vi "CreateSelfReference.vi"(8 "error in (no error)":errorcluster, 11 "XYStage":refnum<class "XYStage.lvclass">) -> (0 "error out":errorcluster, 3 "XYStage out":refnum<class "XYStage.lvclass">)   [LabVIEW 2013, in "XYStage.lvclass"]
doc: "JKI State Machine Objects (SMO) 1.0.0.5\nJKI - JKI\nCopyright (c) 2016, JKI"
uses:
  XYStage.lvclass
  <vilib>/JKI/JKI SMO/SMO/SMO.lvclass
panel:
  # "For instructions on how to use the JKI State Machine Objects, examples and video tutorials, visit:\nhttp://jki.net/state-machine-objects/\n\nJKI State Machine Objects™\nhttp://jki.net/state-machine-objects/\nCopyright (C) 2005-2015, JKI <info@jki.net>\nALL RIGHTS RESERVED"
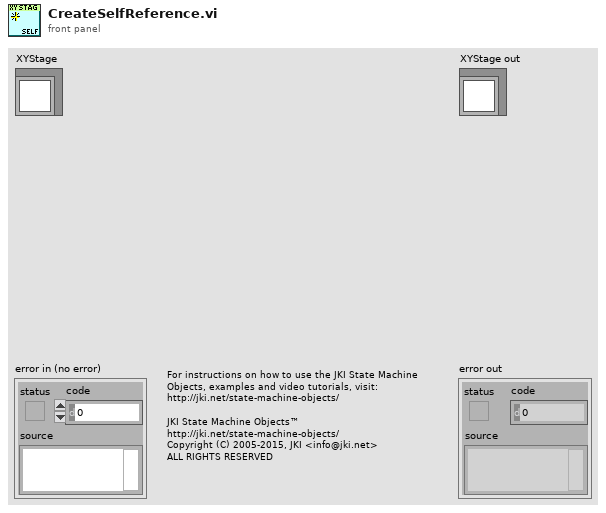
[diagram p1: front panel]
types:
  T1 = typedef "XYStage.lvclass/PrivateData--Ref.ctl" = refnum<data-value>
  T2 = typedef "XYStage.lvclass/PrivateData--Cluster.ctl" = cluster{"Dependencies":T3, "Public Events":T4, "Protected Events":T5, "Private Events":T6, "Configuration":T7, "Target":T8, "Move Parameters":T11}
  T3 = typedef "XYStage.lvclass/Dependencies--Cluster.ctl" = cluster{"Positions":refnum<class "SMO.Dictionary.Variant.lvclass">}
  T4 = typedef "XYStage.lvclass/PublicEvents--Cluster.ctl" = cluster{"MoveComplete":refnum<user-event>, "NewPosition":refnum<user-event>, "UpdatedNamedPosition":refnum<user-event>, "MoveStarted":refnum<user-event>}
  T5 = typedef "XYStage.lvclass/ProtectedEvents--Cluster.ctl" = cluster{"API_Template":refnum<user-event>}
  T6 = typedef "XYStage.lvclass/PrivateEvents--Cluster.ctl" = cluster{"MoveAbsolute":refnum<user-event>, "MoveRelative":refnum<user-event>, "MoveToNamedPosition":refnum<user-event>, "StorePosition":refnum<user-event>, "Home":refnum<user-event>}
  T7 = typedef "XYStage.lvclass/Configuration--Cluster.ctl" = cluster{"Real-World Units":string, "Counts per Unit":dbl}
  T8 = typedef "XYStage.lvclass/TargetPositions--Cluster.ctl" = cluster{"Coords":T9, "Counts":T10}
  T9 = typedef "XYStage.lvclass/(real)Coords--Cluster.ctl" = cluster{"X":dbl, "Y":dbl}
  T10 = typedef "XYStage.lvclass/(counts)Coords--Cluster.ctl" = cluster{"X":i32, "Y":i32}
  T11 = typedef "XYStage.lvclass/MoveParameters--Cluster.ctl" = cluster{"Velocity (units/s)":dbl, "Acceleration (units/s^2)":dbl}
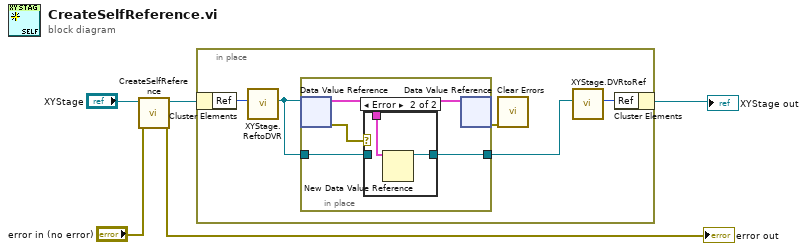
[diagram p0: block diagram]
diagram:
  n1 = call-parent "CreateSelfReference.vi"("error in (no error)"="error in (no error)", "SMO"="XYStage") -> ("error out"=→"error out":errorcluster, "SMO out"=w4:refnum<class "XYStage.lvclass">)  [unwired: 8 in]
  n2 = in-place {
    n3 = in-place-cluster #1(w4) -> ("Ref"=w10:u32)
    n4 = call "XYStage.ReftoDVR.vi"("Ref"=w10) -> ("Ref"=w9:T1)  [unwired: 10 in]
    n5 = in-place {
      in-place-border: [w14] -> w7
      in-place-border: w9 -> [w12]
      n6 = in-place-dvr #2(w9) -> (w11:T2, w13:errorcluster)
      n7 = case shown="Error" w13 {
        tunnel: [w15 w17] -> w14
        tunnel: w12 -> [w15 _]
        tunnel: w11 -> [_ w16]
        frame No Error {
        }
        frame Error {
          n8 = New Data Value Reference(data value=w16) -> (data value reference=w17:refnum<data-value>)  [unwired: 1 in, 1 out]
        }
      }
      n9 = in-place-dvr #2(w11) -> (w6:errorcluster)  [unwired: 1 out]
    }
    n10 = call <vilib>:"Clear Errors.vi"("error in (no error)"=w6) -> ()  [unwired: 5 in, 2 out]
    n11 = call "XYStage.DVRtoRef.vi"("Ref"=w7) -> ("Ref"=w8:u32)  [unwired: 10 in]
    n12 = in-place-cluster #1("Ref"=w8) -> (→"XYStage out":refnum<class "XYStage.lvclass">)
  }
